vi "SWERVE_MODULE_ACQUIRE.vi"(11 "Swerve Module TypDef":T3) -> (0 "Swerve Rotational Speed":dbl, 1 "Swerve Rel Angle":dbl, 2 "Wheel Speed":dbl, 3 "Wheel Distance":dbl, 4 "Swerve Rel Rotation":T2 {"SIN" format="%13.4f"; "COS" format="%13.4f"; "VALUE" format="%13.4f"}, 5 "Swerve Module State":T1={"Speed"=0.0, "Angle"={"VALUE"=0.0, "COS"=1.0, "SIN"=0.0}} {"Angle"."SIN" format="%13.4f"; "Angle"."COS" format="%13.4f"; "Angle"."VALUE" format="%13.4f"})   [LabVIEW 2019]
uses:
  SWERVE_MODULE_TYPDEF.ctl
  <vilib>/Rock Robotics/WPI/MotorControl/WPI_MotorControlDeviceRef.ctl
  <vilib>/Rock Robotics/WPI/MotorControl/WPI_MotorControlType.ctl
  <vilib>/Rock Robotics/SystemInterfaces/DIO/FPGA_DIOPWMChannel.ctl
  <vilib>/Rock Robotics/WPI/PWM/WPI_PWMDeadband.ctl
  <vilib>/Rock Robotics/SystemInterfaces/DIO/FPGA_DIOChannel.ctl
  <vilib>/Rock Robotics/WPI/Encoder/WPI_EncoderDevRef.ctl
  <vilib>/Rock Robotics/SystemInterfaces/Encoder/FPGA_EncoderIdx.ctl
  <vilib>/Rock Robotics/SystemInterfaces/Counter/FPGA_CounterCtrSystemIndex.ctl
  <vilib>/Rock Robotics/WPI/Encoder/WPI_EncoderType.ctl
  <vilib>/Rock Robotics/WPI/ThirdParty/JAS_Junk/TrajLib/ROTATION2D.ctl
  <vilib>/Rock Robotics/WPI/ThirdParty/JAS_Junk/TrajLib/SWERVE_DRIVE_MODULE_STATE.ctl
  <vilib>/Rock Robotics/WPI/ThirdParty/JAS_Junk/TrajLib/Trajectory_Library.lvlib
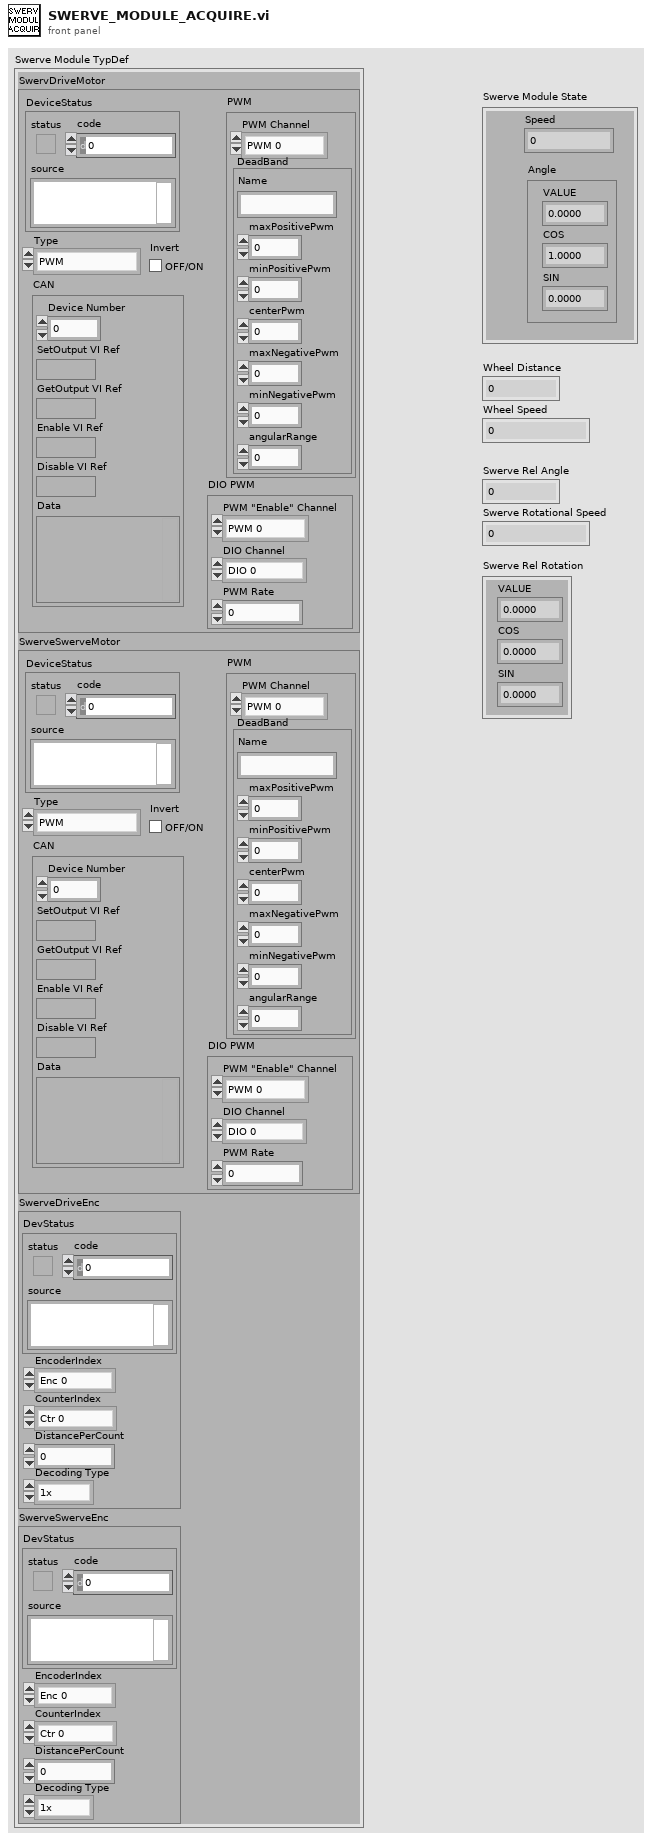
[diagram p1: front panel]
types:
  T1 = typedef "Trajectory_Library.lvlib/SWERVE_DRIVE_MODULE_STATE.ctl" = cluster{"Speed":dbl, "Angle":T2}
  T2 = typedef "Trajectory_Library.lvlib/ROTATION2D.ctl" = cluster{"VALUE":dbl, "COS":dbl, "SIN":dbl}
  T3 = typedef "SWERVE_MODULE_TYPDEF.ctl" = cluster{"SwervDriveMotor":T4, "SwerveSwerveMotor":T4, "SwerveDriveEnc":T9, "SwerveSwerveEnc":T9}
  T4 = typedef "WPI_MotorControlDeviceRef.ctl" = cluster{"DeviceStatus":errorcluster, "Type":T5, "PWM":cluster{"PWM Channel":T6, "DeadBand":T7}, "CAN":cluster{"Device Number":u8, "SetOutput VI Ref":variant, "GetOutput VI Ref":variant, "Enable VI Ref":variant, "Disable VI Ref":variant, "Data":variant}, "Invert":bool, "DIO PWM":cluster{"PWM \"Enable\" Channel":T6, "DIOChannel":T8, "PWM Rate":dbl}}
  T5 = typedef "WPI_MotorControlType.ctl" = enum16{"PWM", "CAN", "DIO PWM"}
  T6 = typedef "FPGA_DIOPWMChannel.ctl" = enum8{"PWM 0", "PWM 1", "PWM 2", "PWM 3", "PWM 4", "PWM 5", "PWM 6", "PWM 7", "PWM 8", "PWM 9", "PWM MXP 0", "PWM MXP 1", "PWM MXP 2", "PWM MXP 3", "PWM MXP 4", "PWM MXP 5", "PWM MXP 6", "PWM MXP 7", "PWM MXP 8", "PWM MXP 9", "Invalid"}
  T7 = typedef "WPI_PWMDeadband.ctl" = cluster{"Name":string, "maxPositivePwm":i32, "minPositivePwm":i32, "centerPwm":i32, "maxNegativePwm":i32, "minNegativePwm":i32, "angularRange":u16}
  T8 = typedef "FPGA_DIOChannel.ctl" = enum8{"DIO 0", "DIO 1", "DIO 2", "DIO 3", "DIO 4", "DIO 5", "DIO 6", "DIO 7", "DIO 8", "DIO 9", "DIO MXP 0", "DIO MXP 1", "DIO MXP 2", "DIO MXP 3", "DIO MXP 4", "DIO MXP 5", "DIO MXP 6", "DIO MXP 7", "DIO MXP 8", "DIO MXP 9", "DIO MXP 10", "DIO MXP 11", "DIO MXP 12", "DIO MXP 13", "DIO MXP 14", "DIO MXP 15", "SPI Port CS1", "SPI Port CS2", "SPI Port CS3", "SPI Port MISO", "SPI Port MOSI", "Invalid"}
  T9 = typedef "WPI_EncoderDevRef.ctl" = cluster{"DevStatus":errorcluster, "EncoderIndex":T10, "CounterIndex":T11, "DistancePerCount":dbl, "Decoding Type":T12}
  T10 = typedef "FPGA_EncoderIdx.ctl" = enum8{"Enc 0", "Enc 1", "Enc 2", "Enc 3", "Enc 4", "Enc 5", "Enc 6", "Enc 7", "Invalid"}
  T11 = typedef "FPGA_CounterCtrSystemIndex.ctl" = enum8{"Ctr 0", "Ctr 1", "Ctr 2", "Ctr 3", "Ctr 4", "Ctr 5", "Ctr 6", "Ctr 7", "Invalid"}
  T12 = typedef "WPI_EncoderType.ctl" = enum16{"1x", "2x", "4x"}
  T13 = typedef "SWERVE_MODULE_MOTOR_CO.ctl" = cluster{"WheelMotorDmd":dbl, "SwerveMotorDmd":dbl}
  T14 = typedef "SWERVE_MODULE_MOTOR_PV.ctl" = cluster{"WheelMotorSpd":dbl, "SwerveMotorSpd":dbl, "WheelDist":dbl, "SwerveAngle":dbl}
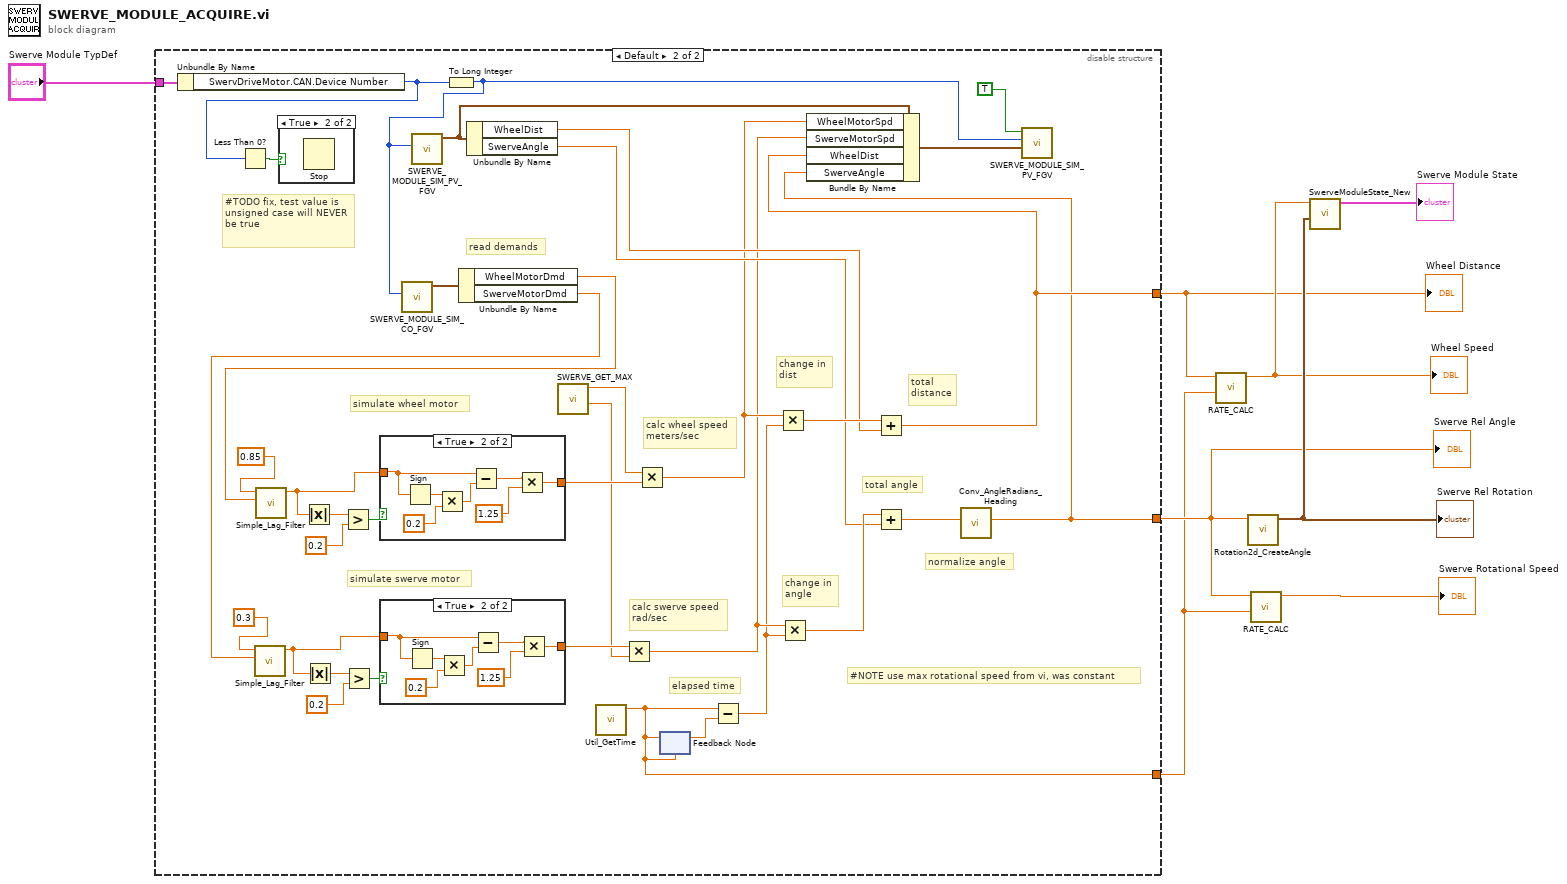
[diagram p0: block diagram]
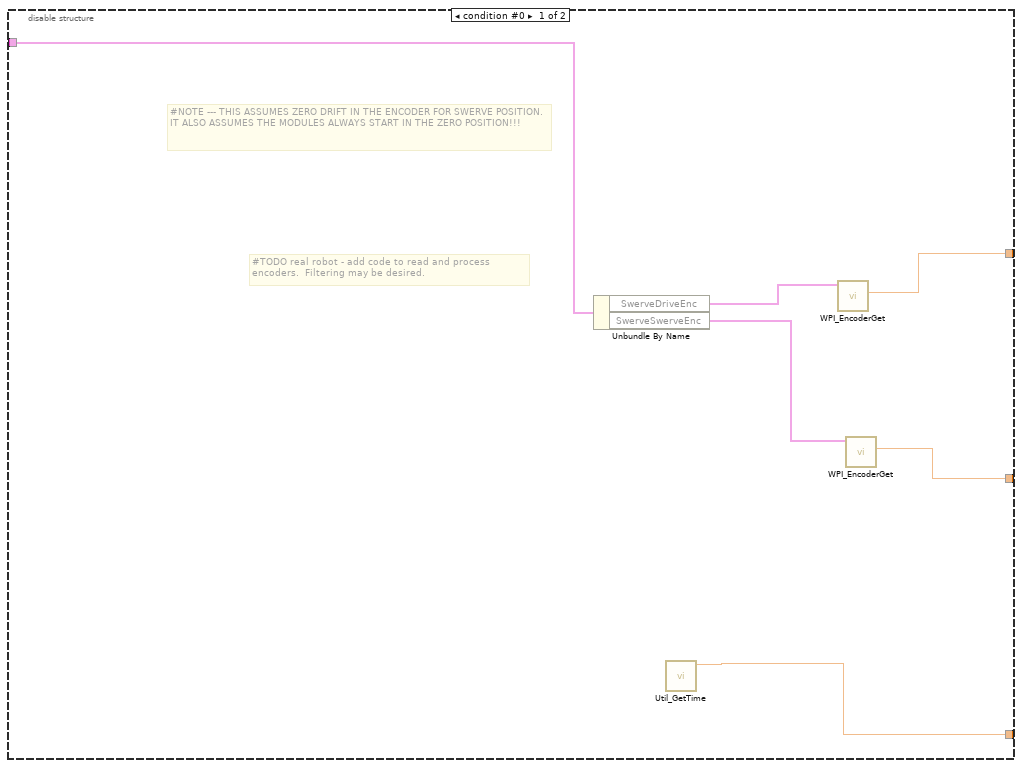
[diagram p2: hidden frame]
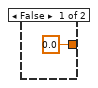
[diagram p3: hidden frame]
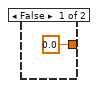
[diagram p4: hidden frame]
diagram:
  n1 = disable-structure shown="Default" {
    disable-tunnel: [w12 w42] -> w4
    disable-tunnel: [w11 w15] -> w2
    disable-tunnel: "Swerve Module TypDef" -> [w10 w50]
    disable-tunnel: [w9 w22] -> w1
    frame condition #0 {
      # "#TODO real robot - add code to read and process encoders.  Filtering may be desired."
      # "#NOTE --- THIS ASSUMES ZERO DRIFT IN THE ENCODER FOR SWERVE POSITION.  IT ALSO ASSUMES THE MODULES ALWAYS START IN THE ZERO POSITION!!!"
      n2 = Unbundle By Name(w10) -> ("SwerveDriveEnc"=w13:T9, "SwerveSwerveEnc"=w14:T9)
      n3 = call <vilib>:"Util_GetTime.vi"() -> ("FPGA_Time_Seconds"=w9:dbl)  [unwired: 10 in, 1 out]
      n4 = call <vilib>:"WPI_EncoderGet.vi"("EncoderDevRef"=w13) -> ("Distance"=w12:dbl)  [unwired: 5 in, 5 out]
      n5 = call <vilib>:"WPI_EncoderGet.vi"("EncoderDevRef"=w14) -> ("Distance"=w11:dbl)  [unwired: 5 in, 5 out]
    }
    frame condition #1 (active) {
      # "normalize angle"
      # "total angle"
      # "total \ndistance"
      # "change in\nangle"
      # "change in\ndist"
      # "calc wheel speed\nmeters/sec"
      # "calc swerve speed\nrad/sec"
      # "simulate swerve motor"
      # "simulate wheel motor"
      # "#NOTE use max rotational speed from vi, was constant"
      # "#TODO fix, test value is unsigned case will NEVER be true"
      # "elapsed time"
      # "read demands"
      n6 = Unbundle By Name(w50) -> ("SwervDriveMotor.CAN.Device Number"=w20:u8)
      n7 = Less Than 0?(x=w20) -> (x < 0?=w38:bool)
      n8 = case shown="True" w38 {
        frame False {
        }
        frame True {
          n9 = Stop() -> ()  [unwired: 1 in]
        }
      }
      n10 = To Long Integer(number=w20) -> (32bit integer=w19:i32)
      n11 = call "SWERVE_MODULE_SIM_CO_FGV.vi"("Index"=w19) -> ("out SwerveModuleMotorDmd"=w41:T13)  [unwired: 10 in]
      n12 = call "SWERVE_MODULE_SIM_PV_FGV.vi"("Index"=w19) -> ("Out SwerveModulePV"=w40:T14)  [unwired: 10 in]
      n13 = Unbundle By Name(w41) -> ("WheelMotorDmd"=w27:dbl, "SwerveMotorDmd"=w34:dbl)
      n14 = call "Simple_Lag_Filter.vi"("Input"=w34, "Lag"=0.3) -> ("Lagged Ouptut"=w33:dbl)  [unwired: 9 in]
      n15 = call "Simple_Lag_Filter.vi"("Input"=w27, "Lag"=0.85) -> ("Lagged Ouptut"=w28:dbl)  [unwired: 9 in]
      n16 = Absolute Value(x=w28) -> (abs(x)=w31:dbl)
      n17 = Absolute Value(x=w33) -> (abs(x)=w37:dbl)
      n18 = Greater?(x=w31, y=0.2) -> (0:w29:bool)
      n19 = Greater?(x=w37, y=0.2) -> (0:w35:bool)
      n20 = case shown="True" w29 {
        tunnel: w28 -> [_ w56]
        tunnel: [0.0 w52] -> w26
        frame False {
        }
        frame True {
          n21 = Sign(1:w56) -> (0:w58:dbl)
          n22 = Multiply(x=w58, y=0.2) -> (x*y=w55:dbl)
          n23 = Subtract(x=w56, y=w55) -> (x-y=w54:dbl)
          n24 = Multiply(x=w54, y=1.25) -> (x*y=w52:dbl)
        }
      }
      n25 = case shown="True" w35 {
        tunnel: w33 -> [_ w64]
        tunnel: [0.0 w60] -> w32
        frame False {
        }
        frame True {
          n26 = Sign(1:w64) -> (0:w66:dbl)
          n27 = Multiply(x=w66, y=0.2) -> (x*y=w63:dbl)
          n28 = Subtract(x=w64, y=w63) -> (x-y=w62:dbl)
          n29 = Multiply(x=w62, y=1.25) -> (x*y=w60:dbl)
        }
      }
      n30 = Unbundle By Name(w40) -> ("WheelDist"=w46:dbl, "SwerveAngle"=w45:dbl)
      n31 = call "SWERVE_GET_MAX.vi"() -> ("Max Rotational Vel (Rad/Sec)"=w21:dbl, "Max Wheel Vel (Meter/Sec)"=w25:dbl)  [unwired: 10 in]
      n32 = call <vilib>:"Util_GetTime.vi"() -> ("FPGA_Time_Seconds"=w22:dbl)  [unwired: 10 in, 1 out]
      n33 = Multiply(x=w32, y=w21) -> (x*y=w43:dbl)
      n34 = Multiply(x=w25, y=w26) -> (x*y=w44:dbl)
      n35 = feedback #1(w22) -> (w24:dbl)
      n36 = feedback-in #1(w22) -> ()
      n37 = Subtract(x=w22, y=w24) -> (x-y=w23:dbl)
      n38 = Multiply(x=w44, y=w23) -> (x*y=w48:dbl)
      n39 = Multiply(x=w43, y=w23) -> (x*y=w49:dbl)
      n40 = Add(x=w48, y=w46) -> (x+y=w42:dbl)
      n41 = Add(x=w49, y=w45) -> (x+y=w16:dbl)
      n42 = call <vilib>:"Conv_AngleRadians_Heading.vi"("Radians"=w16) -> ("Heading"=w15:dbl)  [unwired: 10 in]
      n43 = Bundle By Name(cluster=w40, "WheelMotorSpd"=w44, "SwerveMotorSpd"=w43, "WheelDist"=w42, "SwerveAngle"=w15) -> (w39:T14)
      n44 = call "SWERVE_MODULE_SIM_PV_FGV.vi"("In SwerveModulePV"=w39, "Index"=w19, "WRITE"=TRUE) -> ()  [unwired: 8 in, 1 out]
    }
  }
  "Wheel Distance" <- w4
  "Swerve Rel Angle" <- w2
  n45 = call "RATE_CALC.vi"("Time"=w1, "Input"=w4) -> ("Output"=w5:dbl)  [unwired: 9 in]
  "Wheel Speed" <- w5
  n46 = call <vilib>:"Rotation2d_CreateAngle.vi"("Angle"=w2) -> ("ROTATION"=w7:T2)  [unwired: 10 in]
  "Swerve Rel Rotation" <- w7
  n47 = call "RATE_CALC.vi"("Time"=w1, "Input"=w2) -> ("Output"=→"Swerve Rotational Speed":dbl)  [unwired: 9 in]
  n48 = call <vilib>:"SwerveModuleState_New.vi"("ROTATION"=w7, "Speed"=w5) -> ("SWERVE_DRIVE_MODULE_STATE"=→"Swerve Module State":T1)  [unwired: 9 in]
